vi "Dequeue.vi"(8 "ErrorArray":errorcluster[](array[cluster])) -> (0 "ErrorArray":errorcluster[](array[cluster]), 1 "Data":variant, 2 "Msg":string)   [LabVIEW 2017, in "Bus_class.lvlib" / "Bus.lvclass"]
uses:
  Bus.lvclass
  MsgQueue/Typedef/MsgQueue.ctl
  <vilib>/Utility/error.llb/Error Cluster From Error Code.vi
  <vilib>/ErrorRing/Error Ring.xnode
  <userlib>/NIST/NISTErrorLib/NISTErrorLib.lvlib
  Framework.lvlib
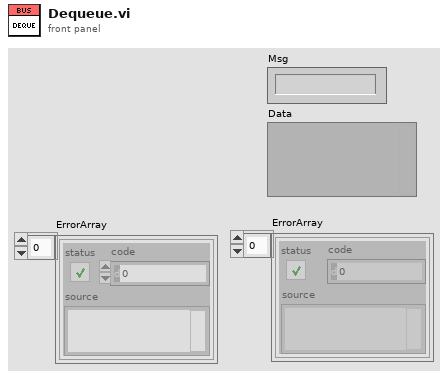
[diagram p1: front panel]
types:
  T1 = typedef "Framework.lvlib/MsgQueue.ctl" = cluster{"Msg":string, "Data":variant}
  T2 = typedef "Framework.lvlib/QueRef.ctl" = refnum<queue>
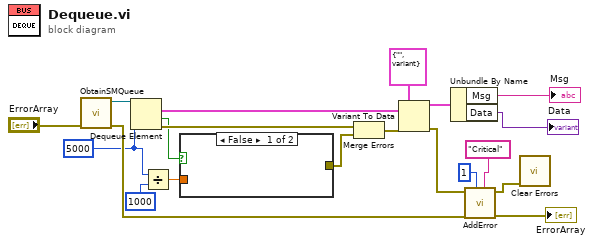
[diagram p0: block diagram]
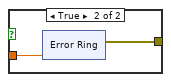
[diagram p2: hidden frame]
diagram:
  w6 = 5000 ("timeout in ms (-1)")
  n1 = call "ObtainSMQueue.vi"("ErrorArray"="ErrorArray") -> ("ErrorArray"=w18:errorcluster[], "QueRef"=w19:T2)  [unwired: 9 in]
  n2 = Dequeue Element(queue=w19, timeout in ms (-1)=w6) -> (element=w15:T1, timed out?=w7:bool, error out=w14:errorcluster)  [unwired: 1 in, 1 out]
  n3 = Divide(x=w6, y=1000) -> (x/y=w4:dbl)
  n4 = case shown="False" w7 {
    tunnel: [_ w22] -> w2
    tunnel: w4 -> [_ w21]
    frame False {
    }
    frame True {
      n5 = xnode "Error Ring"("parameter 0"=w21) -> ("error out"=w22:errorcluster)
    }
  }
  n6 = Merge Errors(w14, w2) -> (w3:errorcluster)
  n7 = Variant To Data(error in=w3, type=T1 {"Msg"="", "Data"=variant} ("MsgQueue"), Variant=w15) -> (data=w12:T1, error out=w8:errorcluster)
  n8 = Unbundle By Name(w12) -> ("Msg"=→"Msg":string, "Data"=→"Data":variant)
  n9 = call <userlib>:"AddError.vi"("Severity"="Critical", "Priority"=u8 1, "ErrorArray"=w18, "error in (no error)"=w8) -> ("ErrorArray"=→"ErrorArray":errorcluster[], "error out"=w1:errorcluster)  [unwired: 6 in]
  n10 = call <vilib>:"Clear Errors.vi"("error in (no error)"=w1) -> ()  [unwired: 5 in, 2 out]
